vi "Send Console Reply Msg.vi"(8 "error in (no error)":errorcluster, 10 "Console Reply":refnum<class "Console Reply.lvclass">, 11 "Console in":refnum<class "Console.lvclass">) -> (0 "error out":errorcluster, 3 "Console out":refnum<class "Console.lvclass">)   [LabVIEW 2015, in "EditPanel API.lvlib" / "Console.lvclass"]
uses:
  Console.lvclass
  Console Reply/Console Reply/Console Reply.lvclass
  Type Definition/Console_Q Data Type.ctl
  Panel Control_Interface/Panel_interface/Panel Controller Interface.lvclass
  Console.lvclass/Console.ctl
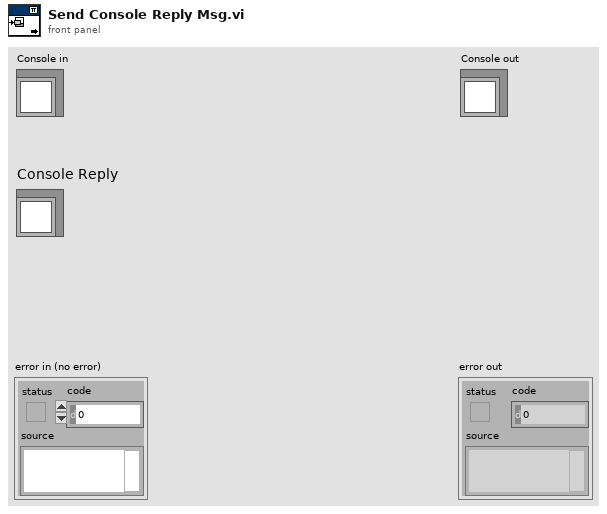
[diagram p1: front panel]
types:
  T1 = typedef "EditPanel API.lvlib/Console.lvclass/Console_Q Data Type.ctl" = cluster{"Console Reply":refnum<class "Console Reply.lvclass">, "Panel":refnum<class "Panel Controller Interface.lvclass">}
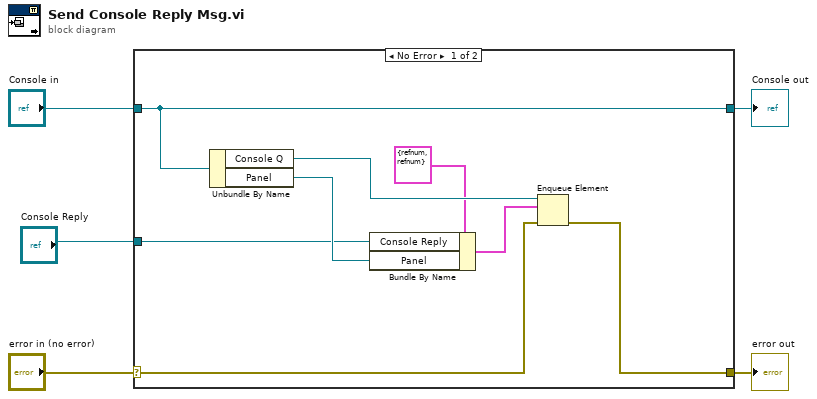
[diagram p0: block diagram]
diagram:
  n1 = case shown="No Error" "error in (no error)" {
    selector: "error in (no error)" -> [w11 w15]
    tunnel: [w10 w15] -> w4
    tunnel: [w13 w14] -> w2
    tunnel: "Console in" -> [w13 w14]
    tunnel: "Console Reply" -> [w6 _]
    frame No Error {
      n2 = Unbundle By Name(w13) -> ("Console Q"=w12:refnum<queue>, "Panel"=w8:refnum<class "Panel Controller Interface.lvclass">)
      n3 = Bundle By Name(cluster=T1 {"Console Reply"=refnum, "Panel"=refnum} ("element"), "Console Reply"=w6, "Panel"=w8) -> (w7:T1)
      n4 = Enqueue Element(queue=w12, element=w7, error in (no error)=w11) -> (error out=w10:errorcluster)  [unwired: 1 in, 2 out]
    }
    frame Error {
    }
  }
  "error out" <- w4
  "Console out" <- w2
